vi "Create File.vi"(8 "error in":errorcluster, 11 "Root Path":path) -> (0 "error out":errorcluster, 1 "File path out":path, 3 "refnum out":refnum<file>)   [LabVIEW 2021]
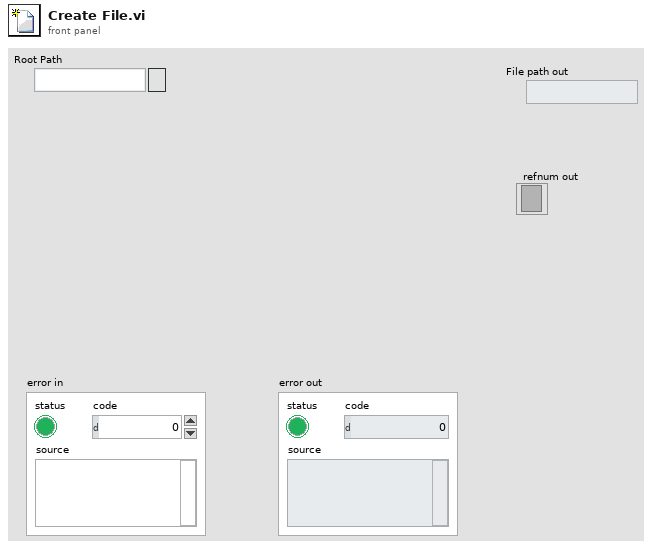
[diagram p1: front panel]
types:
  T1 = enum16{"open", "replace", "create", "open or create", "replace or create", "replace or create with confirmation"}
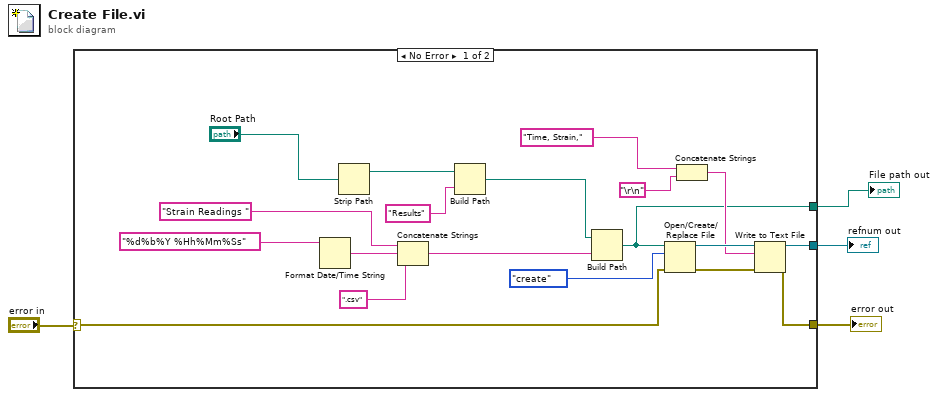
[diagram p0: block diagram]
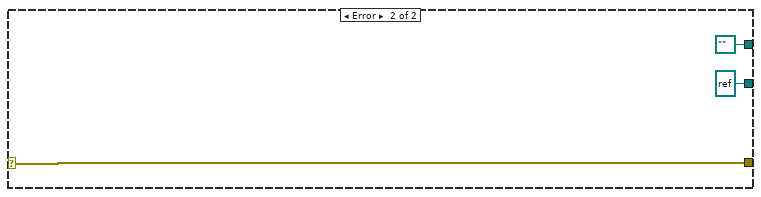
[diagram p2: hidden frame]
diagram:
  n1 = case shown="No Error" "error in" {
    selector: "error in" -> [w9 w26]
    tunnel: [w8 w26] -> w3
    tunnel: [w7 refnum<file> refnum ("refnum out")] -> w2
    tunnel: [w5 path "" ("appended path")] -> w1
    frame No Error {
      n2 = Format Date/Time String(time format string (%c)="%d%b%Y %Hh%Mm%Ss") -> (date/time string=w22:string)  [unwired: 2 in]
      n3 = Strip Path(path="Root Path") -> (stripped path=w10:path)  [unwired: 1 out]
      n4 = Concatenate Strings("Strain Readings " ("string"), w22, ".csv" ("string")) -> (w20:string)
      n5 = Build Path(base path=w10, name or relative path="Results") -> (appended path=w19:path)
      n6 = Build Path(base path=w19, name or relative path=w20) -> (appended path=w5:path)
      n7 = Open/Create/Replace File(file path (use dialog)=w5, error in=w9, operation (0:open)=T1."create") -> (refnum out=w17:refnum<file>, error out=w16:errorcluster)  [unwired: 3 in, 1 out]
      n8 = Concatenate Strings("Time, Strain,", "\r\n") -> (w13:string)
      n9 = Write to Text File(file (use dialog)=w17, text=w13, error in=w16) -> (refnum out=w7:refnum<file>, error out=w8:errorcluster)  [unwired: 1 in, 1 out]
    }
    frame Error {
    }
  }
  "error out" <- w3
  "refnum out" <- w2
  "File path out" <- w1
